vi "Write Kamikaze DVR.vi"(8 "error in (no error)":errorcluster, 10 "Kamikaze DVR":T1, 11 "Mother in":refnum<class "Mother.lvclass">) -> (0 "error out":errorcluster, 3 "Mother out":refnum<class "Mother.lvclass">)   [LabVIEW 2014, in "Mother.lvclass"]
uses:
  Mother.lvclass
  Kamikaze DVR.ctl
  Mother.lvclass/Mother.ctl
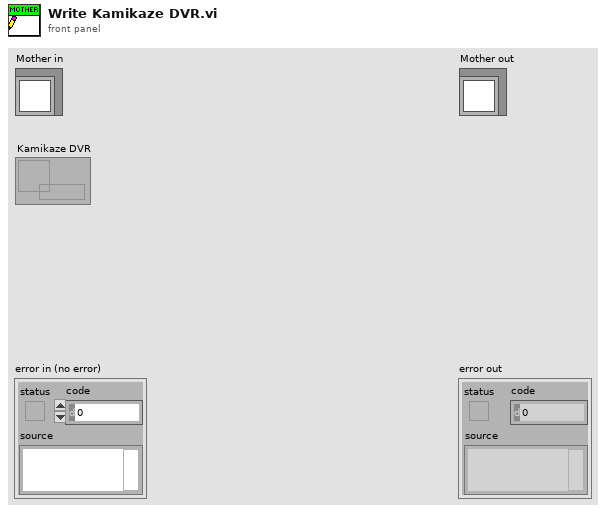
[diagram p1: front panel]
types:
  T1 = typedef "Kamikaze DVR.ctl" = refnum<data-value>
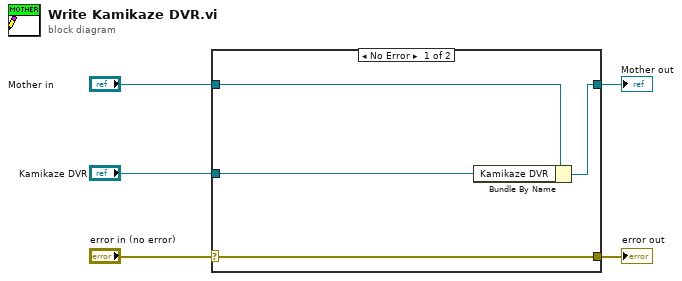
[diagram p0: block diagram]
diagram:
  n1 = case shown="No Error" "error in (no error)" {
    selector: "error in (no error)" -> [w9 w10]
    tunnel: [w9 w10] -> w4
    tunnel: [w7 w11] -> w2
    tunnel: "Mother in" -> [w8 w11]
    tunnel: "Kamikaze DVR" -> [w6 _]
    frame No Error {
      n2 = Bundle By Name(cluster=w8, "Kamikaze DVR"=w6) -> (w7:refnum<class "Mother.lvclass">)
    }
    frame Error {
    }
  }
  "error out" <- w4
  "Mother out" <- w2
